vi "Name_check_login.vi"(9 "LAST NAME:":string, 10 "NAME:":string, 11 "Boolean":bool) -> (3 "OK":bool)   [LabVIEW 2016]
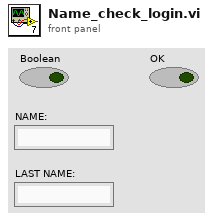
[diagram p1: front panel]
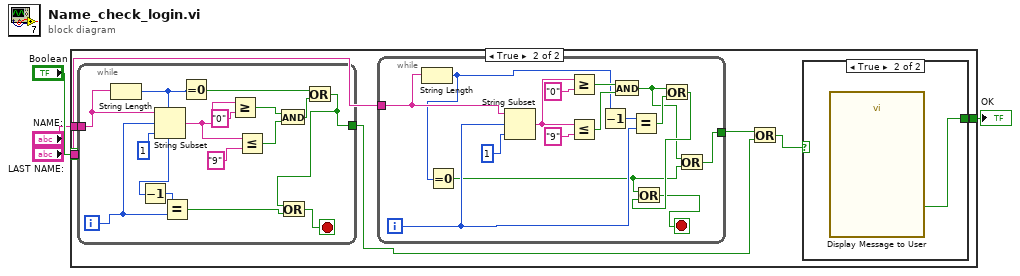
[diagram p0: block diagram]
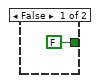
[diagram p2: hidden frame]
diagram:
  n1 = case shown="True" "Boolean" {
    tunnel: "NAME:" -> [_ w11]
    tunnel: "LAST NAME:" -> [_ w10]
    tunnel: [FALSE ("OK") w6] -> w4
    frame False {
    }
    frame True {
      n2 = while {
        tunnel: w11 -> [w43]
        tunnel: [w32] -> w8
        i -> [w30]
        stop <- w36 stop-if-true
        n3 = String Length(string=w43) -> (length=w35:i32)
        n4 = Decrement(x=w35) -> (x-1=w44:i32)
        n5 = String Subset(string=w43, offset (0)=w30, length (rest)=1 ("offset (0)")) -> (substring=w40:string)
        n6 = Equal?(x=w44, y=w30) -> (x = y?=w37:bool)
        n7 = Equal To 0?(x=w35) -> (x = 0?=w33:bool)
        n8 = Greater Or Equal?(x=w40, y="0") -> (x >= y?=w39:bool)
        n9 = Less Or Equal?(x=w40, y="9") -> (x <= y?=w38:bool)
        n10 = And(x=w39, y=w38) -> (x .and. y?=w34:bool)
        n11 = Or(x=w33, y=w34) -> (x .or. y?=w32:bool)
        n12 = Or(x=w32, y=w37) -> (x .or. y?=w36:bool)
      }
      n13 = while {
        tunnel: w10 -> [w20]
        tunnel: [w12] -> w9
        i -> [w17]
        stop <- w15 stop-if-true
        n14 = String Length(string=w20) -> (length=w19:i32)
        n15 = Equal To 0?(x=w19) -> (x = 0?=w13:bool)
        n16 = String Subset(string=w20, offset (0)=w17, length (rest)=1 ("offset (0)")) -> (substring=w24:string)
        n17 = Greater Or Equal?(x=w24, y="0") -> (x >= y?=w25:bool)
        n18 = Less Or Equal?(x=w24, y="9") -> (x <= y?=w26:bool)
        n19 = Decrement(x=w19) -> (x-1=w21:i32)
        n20 = And(x=w25, y=w26) -> (x .and. y?=w14:bool)
        n21 = Equal?(x=w21, y=w17) -> (x = y?=w27:bool)
        n22 = Or(x=w14, y=w27) -> (x .or. y?=w18:bool)
        n23 = Or(x=w13, y=w18) -> (x .or. y?=w15:bool)
        n24 = Or(x=w14, y=w13) -> (x .or. y?=w12:bool)
      }
      n25 = Or(x=w9, y=w8) -> (x .or. y?=w7:bool)
      n26 = case shown="True" w7 {
        selector: w7 -> [w28 _]
        tunnel: [w28 w29] -> w6
        frame False {
        }
        frame True {
          n27 = call "Display Message to User"() -> ("OK"=w29:bool)  [unwired: 10 in, 1 out]
        }
      }
    }
  }
  "OK" <- w4
